vi "Write Report Generator.vi"(8 "error in (no error)":errorcluster, 10 "Report Generator":refnum<class "Report Generator.lvclass">, 11 "Report In":refnum<class "Report.lvclass">) -> (0 "error out":errorcluster, 3 "Report Out":refnum<class "Report.lvclass">)   [LabVIEW 2020, in "Reports.lvlib" / "Report.lvclass"]
uses:
  Report.lvclass
  Report Generator/Report Generator.lvclass
  Report.lvclass/Report.ctl
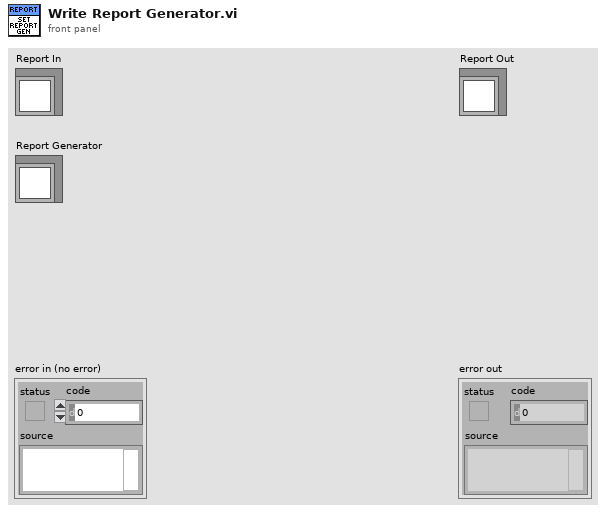
[diagram p1: front panel]
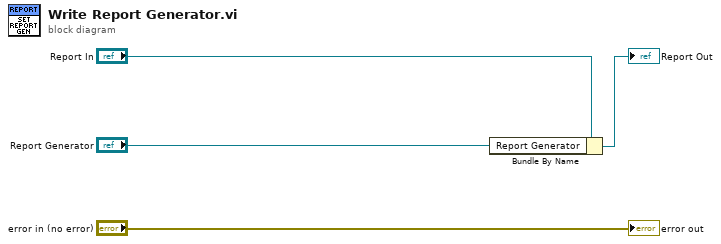
[diagram p0: block diagram]
diagram:
  n1 = Bundle By Name(cluster="Report In", "Report Generator"="Report Generator") -> (→"Report Out":refnum<class "Report.lvclass">)
  "error out" <- "error in (no error)"
